vi "边沿计数(外时钟).vi"() -> ()   [LabVIEW 2013]
doc: "This example demonstrates how to count the pulse's edges."
uses:
  <userlib>/ArtDAQ/_SubVI/ArtDAQ_CreateCICountEdgesChan.vi
  <userlib>/ArtDAQ/_SubVI/ArtDAQ_CfgSampClkTiming.vi
  <userlib>/ArtDAQ/_SubVI/ArtDAQ_Read Counter U32 NSamp.vi
panel:
  in  "每通道点数":i32=100
  in  "采样速率":dbl=10000.0 format="%#_13g"
  in  "时钟源":string="/Dev1/PFI3"
  in  "计数器":string="Dev1/CTR0"
  out "数据":u32[](array[numeric])
  in  "停止":bool
  out "错误输出":errorcluster
  # "通道属性"
  # "定时"
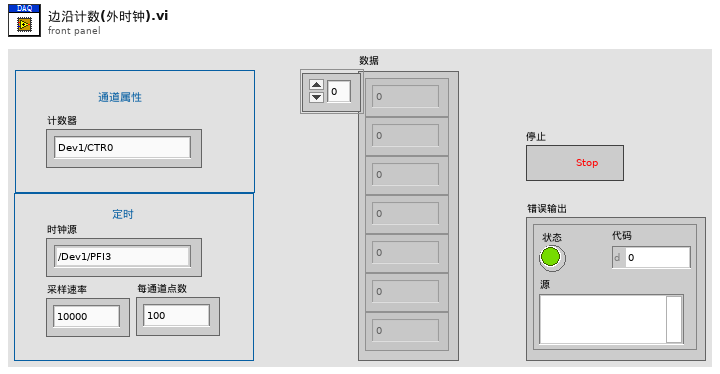
[diagram p1: front panel]
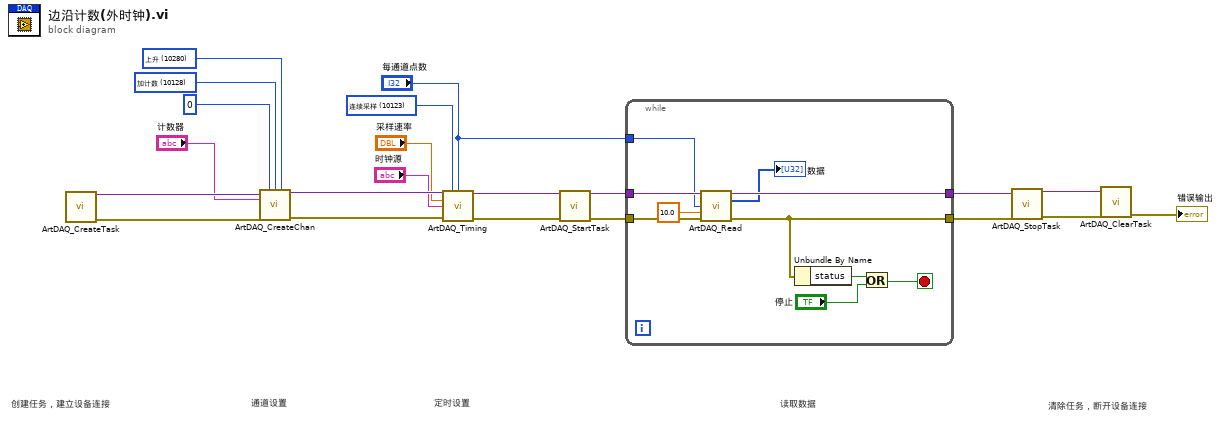
[diagram p0: block diagram]
diagram:
  w2 = 10123 items=["有限点采样"=10178, "连续采样"=10123] ("SampleMode")
  w17 = 10280 items=["上升"=10280, "下降"=10171] ("Edge")
  w18 = 10128 items=["加计数"=10128, "减计数"=10124, "外部控制"=10326] ("CountDir")
  # "清除任务，断开设备连接"
  # "读取数据"
  # "定时设置"
  # "通道设置"
  # "创建任务，建立设备连接"
  n1 = call <userlib>:"ArtDAQ_CreateTask.vi"() -> ("任务句柄"=w21:variant, "错误输出"=w20:errorcluster)  [unwired: 14 in]
  n2 = call-poly <userlib>:"ArtDAQ_CreateChan.vi"("任务句柄"=w21, "初始计数"=u32 0 ("InitialCount"), "计数方向"=w18, "边沿"=w17, "计数器"="计数器", "错误输入"=w20) -> ("任务句柄"=w8:variant, "错误输出"=w6:errorcluster)  [unwired: 8 in]
  n3 = call-poly <userlib>:"ArtDAQ_Timing.vi"("任务句柄"=w8, "采样模式"=w2, "每通道采样数"="每通道点数", "采样率"="采样速率", "源"="时钟源", "错误输入"=w6) -> ("任务句柄"=w7:variant, "错误输出"=w5:errorcluster)  [unwired: 8 in]
  n4 = call <userlib>:"ArtDAQ_StartTask.vi"("任务句柄"=w7, "错误输入"=w5) -> ("任务句柄"=w10:variant, "错误输出"=w9:errorcluster)  [unwired: 12 in]
  n5 = while {
    tunnel: [w31] -> w15
    tunnel: [w27] -> w13
    tunnel: w10 -> [w30]
    tunnel: w9 -> [w29]
    tunnel: "每通道点数" -> [w23]
    stop <- w24 stop-if-true
    n6 = call-poly <userlib>:"ArtDAQ_Read.vi"("任务句柄"=w30, "每通道采样数"=w23, "超时s"=10.0 ("Timeout"), "错误输入"=w29) -> ("任务句柄"=w31:variant, "数据"=→"数据":u32[], "错误输出"=w27:errorcluster)  [unwired: 9 in]
    n7 = Unbundle By Name(w27) -> ("status"=w26:bool)
    n8 = Or(x=w26, y="停止") -> (x .or. y?=w24:bool)
  }
  n9 = call <userlib>:"ArtDAQ_StopTask.vi"("任务句柄"=w15, "错误输入"=w13) -> ("任务句柄"=w14:variant, "错误输出"=w12:errorcluster)  [unwired: 12 in]
  n10 = call <userlib>:"ArtDAQ_ClearTask.vi"("任务句柄"=w14, "错误输入"=w12) -> ("错误输出"=→"错误输出":errorcluster)  [unwired: 13 in]
